vi "pythonHyperstack.vi"(1 "refresh_time":dbl=0.1, 2 "image reference":refnum<data-value>) -> (0 "return type":dbl)   [LabVIEW 2017]
uses:
  globalUtilities.vi
  dll/wormUtilities/x64/Release/wormUtilities.dll
panel:
  out "out":sgl[](array[numeric])
  out "displayStop":bool
  out "Numeric":i32
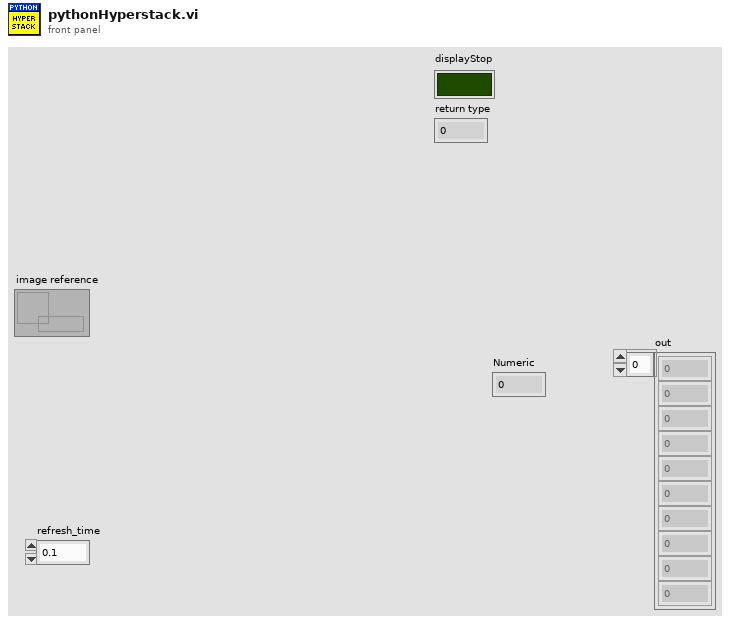
[diagram p1: front panel]
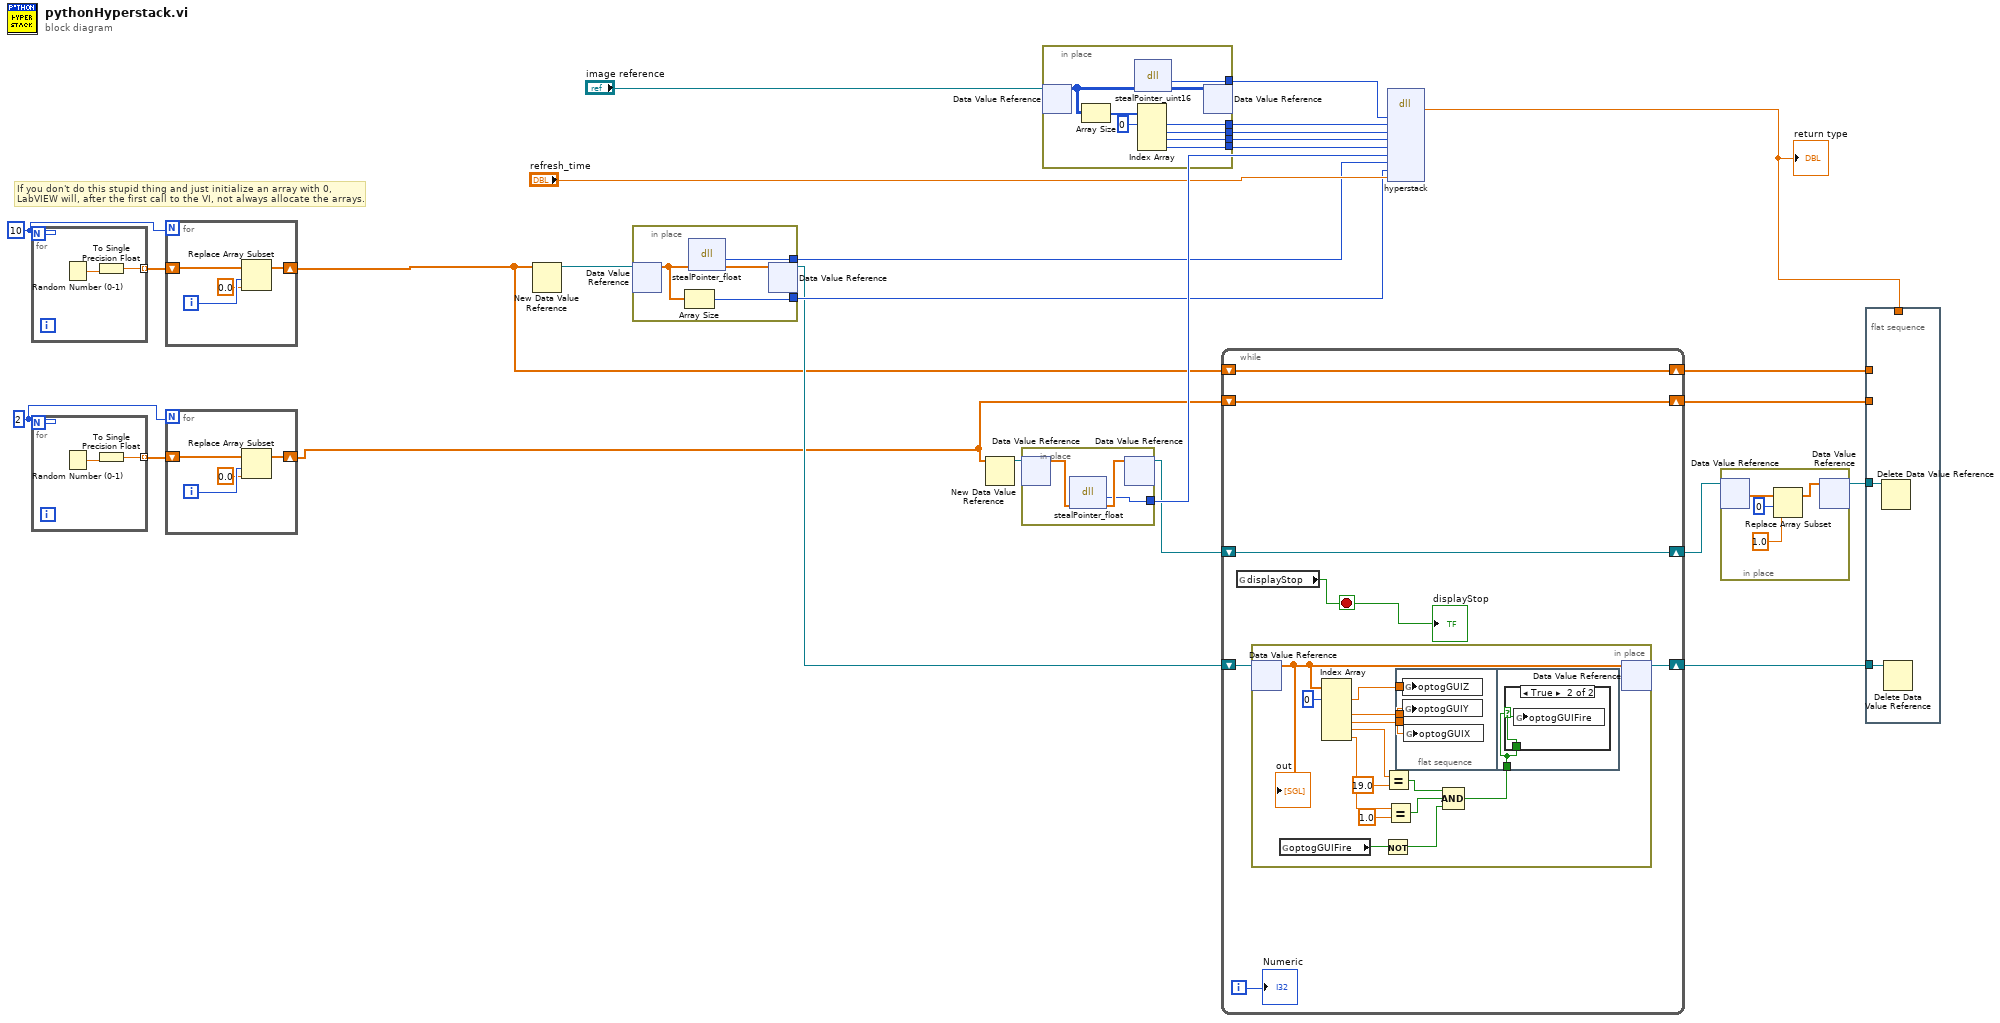
[diagram p0: block diagram]
diagram:
  w5 = 2
  w4 = 10
  # "If you don't do this stupid thing and just initialize an array with 0, \nLabVIEW will, after the first call to the VI, not always allocate the arrays."
  n1 = for {
    N: w4 -> [_]
    tunnel: [w27] -> w9 mode=indexing
    n2 = Random Number (0-1)() -> (number: 0 to 1=w28:dbl)
    n3 = To Single Precision Float(number=w28) -> (single precision float=w27:sgl)
  }
  n4 = for {
    N: w5 -> [_]
    tunnel: [w29] -> w7 mode=indexing
    n5 = Random Number (0-1)() -> (number: 0 to 1=w30:dbl)
    n6 = To Single Precision Float(number=w30) -> (single precision float=w29:sgl)
  }
  n7 = for {
    N: w4 -> [_]
    shift-right: [w31] -> w8
    shift-left: w9 -> [w34]
    i -> [w33]
    n8 = Replace Array Subset(array=w34, new element=sgl 0.0 ("new element/subarray"), index=w33) -> (w31:sgl[])
  }
  n9 = for {
    N: w5 -> [_]
    shift-right: [w35] -> w6
    shift-left: w7 -> [w38]
    i -> [w37]
    n10 = Replace Array Subset(array=w38, new element=sgl 0.0 ("new element/subarray"), index=w37) -> (w35:sgl[])
  }
  n11 = New Data Value Reference(data value=w8) -> (data value reference=w13:refnum<data-value>)  [unwired: 1 in, 1 out]
  n12 = in-place {
    in-place-border: [w41] -> w21
    in-place-border: [w39] -> w20
    n13 = in-place-dvr #1(w13) -> (w40:sgl[])  [unwired: 1 out]
    n14 = Array Size(array=w40) -> (size(s)=w39:i32)
    n15 = dll-call lib="C:/Users/francesco/dev/pump-probe/dll/wormUtilities/x64/Release/wormUtilities.dll" fn="stealPointer_float"("A"=w40) -> ("return type"=w41:i64, "A"=w42:sgl[])  [unwired: 3 in, 2 out]
    n16 = in-place-dvr #1(w42) -> (w11:refnum<data-value>)  [unwired: 1 out]
  }
  n17 = New Data Value Reference(data value=w6) -> (data value reference=w25:refnum<data-value>)  [unwired: 1 in, 1 out]
  n18 = in-place {
    in-place-border: [w43] -> w26
    n19 = in-place-dvr #2(w25) -> (w44:sgl[])  [unwired: 1 out]
    n20 = dll-call lib="C:/Users/francesco/dev/pump-probe/dll/wormUtilities/x64/Release/wormUtilities.dll" fn="stealPointer_float"("A"=w44) -> ("return type"=w43:i64, "A"=w45:sgl[])  [unwired: 3 in, 2 out]
    n21 = in-place-dvr #2(w45) -> (w24:refnum<data-value>)  [unwired: 1 out]
  }
  n22 = in-place {
    in-place-border: [w54] -> w18
    in-place-border: [w49] -> w17
    in-place-border: [w48] -> w16
    in-place-border: [w47] -> w15
    in-place-border: [w46] -> w14
    n23 = in-place-dvr #3("image reference") -> (w51:u16[][][][])  [unwired: 1 out]
    n24 = Array Size(array=w51) -> (size(s)=w53:i32[])
    n25 = dll-call lib="C:/Users/francesco/dev/pump-probe/dll/wormUtilities/x64/Release/wormUtilities.dll" fn="stealPointer_uint16"("A"=w51) -> ("return type"=w54:i64, "A"=w50:u16[][][][])  [unwired: 3 in, 2 out]
    n26 = Index Array(array=w53, index #1=0 ("index")) -> (element #1=w49:i32, element #2=w48:i32, element #3=w47:i32, element #4=w46:i32)  [unwired: 3 in]
    n27 = in-place-dvr #3(w50) -> ()  [unwired: 2 out]
  }
  n28 = while {
    shift-right: [w57] -> w12
    shift-left: w11 -> [w59]
    shift-right: [w60] -> w23
    shift-left: w24 -> [w60]
    shift-right: [w56] -> w2
    shift-left: w8 -> [w56]
    shift-right: [w55] -> w1
    shift-left: w6 -> [w55]
    i -> [w58]
    stop <- w61 stop-if-true
    n29 = global read "globalUtilities.vi" "displayStop"() -> (w61:bool)
    "displayStop" <- w61
    n30 = in-place {
      n31 = in-place-dvr #4(w59) -> (w75:sgl[])  [unwired: 1 out]
      "out" <- w75
      n32 = global read "globalUtilities.vi" "optogGUIFire"() -> (w64:bool)
      n33 = Index Array(array=w75, index #1=0 ("index")) -> (element #1=w73:sgl, element #3=w72:sgl, element #4=w71:sgl, element #5=w70:sgl, element #6=w68:sgl)  [unwired: 5 in, 1 out]
      n34 = Not(x=w64) -> (.not. x?=w62:bool)
      n35 = Equal?(x=w70, y=sgl 19.0) -> (x = y?=w66:bool)
      n36 = Equal?(x=w68, y=sgl 1.0) -> (x = y?=w65:bool)
      n37 = flat-sequence {
        tunnel: w73 -> [w78]
        tunnel: w72 -> [w77]
        tunnel: w71 -> [w76]
        tunnel: w63 -> [w79]
        frame #0 {
          n38 = global write "globalUtilities.vi" "optogGUIZ"(w78) -> ()
          n39 = global write "globalUtilities.vi" "optogGUIY"(w77) -> ()
          n40 = global write "globalUtilities.vi" "optogGUIX"(w76) -> ()
        }
        frame #1 {
          n41 = case shown="True" w79 {
            tunnel: w79 -> [_ w80]
            frame False {
            }
            frame True {
              n42 = global write "globalUtilities.vi" "optogGUIFire"(w80) -> ()
            }
          }
        }
      }
      n43 = Compound Arithmetic op=AND(w66, w65, w62) -> (w63:bool)
      n44 = in-place-dvr #4(w75) -> (w57:refnum<data-value>)  [unwired: 1 out]
    }
    "Numeric" <- w58
  }
  n45 = dll-call lib="C:/Users/francesco/dev/pump-probe/dll/wormUtilities/x64/Release/wormUtilities.dll" fn="hyperstack"("A"=w18, "shape0"=w17, "shape1"=w16, "shape2"=w15, "shape3"=w14, "stop"=w26, "out"=w21, "out_n"=w20, "refresh_time"="refresh_time") -> ("return type"=w3:dbl)  [unwired: 12 in, 2 out]
  "return type" <- w3
  n46 = in-place {
    n47 = in-place-dvr #5(w23) -> (w84:sgl[])  [unwired: 1 out]
    n48 = Replace Array Subset(array=w84, new element=sgl 1.0 ("new element/subarray"), index=0) -> (w81:sgl[])
    n49 = in-place-dvr #5(w81) -> (w10:refnum<data-value>)  [unwired: 1 out]
  }
  n50 = flat-sequence {
    tunnel: w12 -> [w86]
    tunnel: w10 -> [w85]
    tunnel: w3 -> [_]
    tunnel: w2 -> [_]
    tunnel: w1 -> [_]
    frame #0 {
      n51 = Delete Data Value Reference(data value reference=w85) -> ()  [unwired: 1 in, 2 out]
      n52 = Delete Data Value Reference(data value reference=w86) -> ()  [unwired: 1 in, 2 out]
    }
  }
